vi "Trigger Pulse.vi"() -> ()   [LabVIEW 2015]
uses:
  <vilib>/DAQmx/write.llb/DAQmx Write (Digital Bool 1Line 1Point).vi
  <vilib>/DAQmx/create/channels.llb/DAQmx Create Channel (DO-Digital Output).vi
  <vilib>/DAQmx/miscellaneous.llb/DAQmx Fill In Error Info.vi
panel:
  in  "milliseconds duration":u32=10
  in  "lines":tag="Dev1/port1/line1"
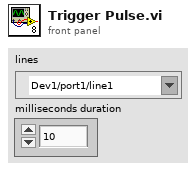
[diagram p1: front panel]
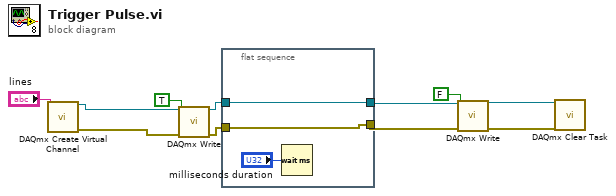
[diagram p0: block diagram]
diagram:
  n1 = call-poly <vilib>:"DAQmx Create Virtual Channel.vi"("lines"="lines") -> ("task out"=w10:refnum<k21>, "error out"=w9:errorcluster)  [unwired: 13 in]
  n2 = call-poly <vilib>:"DAQmx Write.vi"("task/channels in"=w10, "data"=TRUE, "error in"=w9) -> ("task out"=w6:refnum<k21>, "error out"=w7:errorcluster)  [unwired: 10 in, 1 out]
  n3 = flat-sequence {
    tunnel: w7 -> [w12]
    tunnel: w6 -> [w13]
    tunnel: [w13] -> w4
    tunnel: [w12] -> w5
    frame #0 {
      n4 = Wait (ms)(milliseconds to wait="milliseconds duration") -> ()  [unwired: 1 out]
    }
  }
  n5 = call-poly <vilib>:"DAQmx Write.vi"("task/channels in"=w4, "data"=FALSE, "error in"=w5) -> ("task out"=w1:refnum<k21>, "error out"=w2:errorcluster)  [unwired: 10 in, 1 out]
  n6 = call <vilib>:"DAQmx Clear Task.vi"("task in"=w1, "error in"=w2) -> ()  [unwired: 13 in, 1 out]
